vi "AcquireWaveformFromOscill.vi"(4 "error in":errorcluster, 5 "byte count":u32=15000, 6 "Channel (1: Channel 1)":u16(ring)=1 items=["Channel 1"=1, "Channel 2"=2, "Channel 3"=3, "Channel 4"=4], 7 "VISA resource name":refnum<visa-resource-name>) -> (0 "error out":errorcluster, 1 "Number of points":dbl, 2 "Numeric":dbl, 3 "Waveform Graph":waveform(dbl)(graph))   [LabVIEW 2013]
panel:
  out "read buffer":string
  out "Xref":dbl
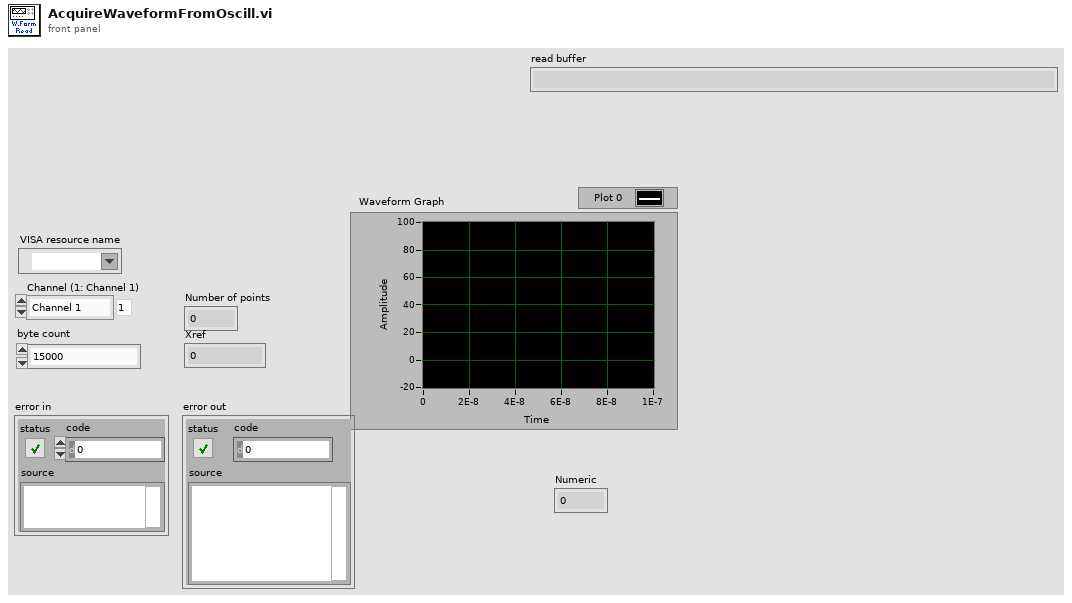
[diagram p1: front panel]
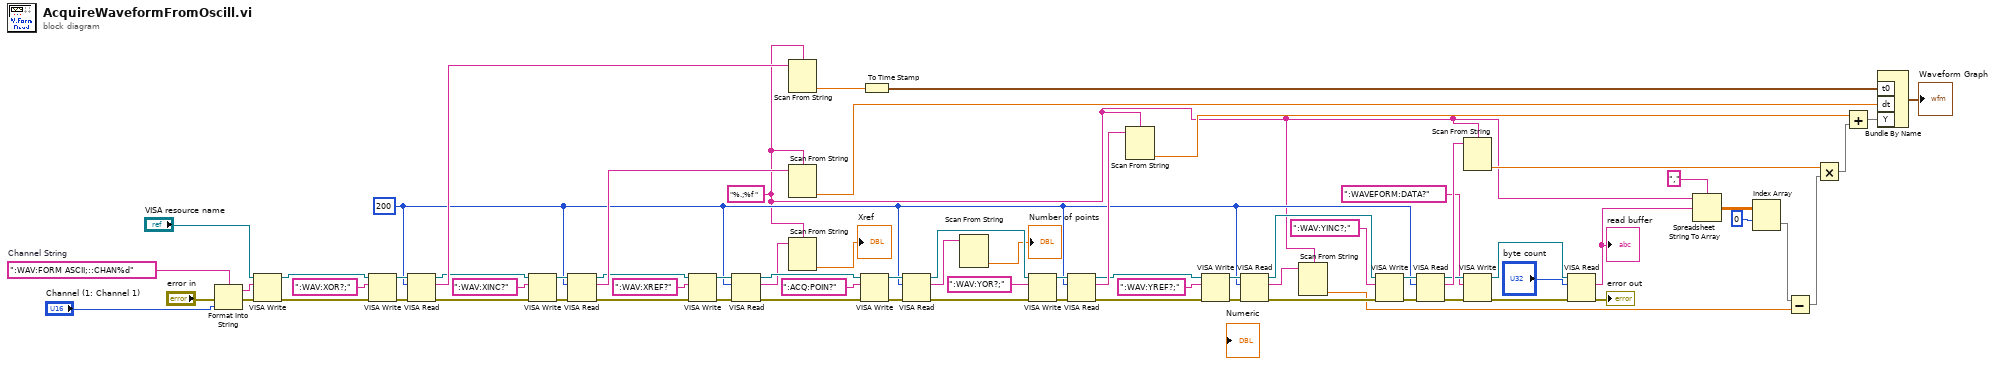
[diagram p0: block diagram]
diagram:
  w9 = ":WAV:FORM ASCII;::CHAN%d"  # Channel String
  w37 = u32 200 ("byte count")
  w12 = "%.;%f " ("format string")
  n1 = Format Into String(format string=w9, error in="error in", "Channel (1: Channel 1)") -> (resulting string=w8:string, error out=w6:errorcluster)  [unwired: 1 in]
  n2 = VISA Write(VISA resource name="VISA resource name", write buffer=w8, error in (no error)=w6) -> (VISA resource name out=w15:refnum<visa-resource-name>, error out=w14:errorcluster)  [unwired: 1 out]
  n3 = VISA Write(VISA resource name=w15, write buffer=":WAV:XOR?;", error in (no error)=w14) -> (VISA resource name out=w74:refnum<visa-resource-name>, error out=w73:errorcluster)  [unwired: 1 out]
  n4 = VISA Read(VISA resource name=w74, byte count=w37, error in (no error)=w73) -> (VISA resource name out=w69:refnum<visa-resource-name>, read buffer=w71:string, error out=w70:errorcluster)  [unwired: 1 out]
  n5 = VISA Write(VISA resource name=w69, write buffer=":WAV:XINC?", error in (no error)=w70) -> (VISA resource name out=w68:refnum<visa-resource-name>, error out=w67:errorcluster)  [unwired: 1 out]
  n6 = VISA Read(VISA resource name=w68, byte count=w37, error in (no error)=w67) -> (VISA resource name out=w55:refnum<visa-resource-name>, read buffer=w66:string, error out=w53:errorcluster)  [unwired: 1 out]
  n7 = VISA Write(VISA resource name=w55, write buffer=":WAV:XREF?", error in (no error)=w53) -> (VISA resource name out=w54:refnum<visa-resource-name>, error out=w52:errorcluster)  [unwired: 1 out]
  n8 = VISA Read(VISA resource name=w54, byte count=w37, error in (no error)=w52) -> (VISA resource name out=w51:refnum<visa-resource-name>, read buffer=w47:string, error out=w50:errorcluster)  [unwired: 1 out]
  n9 = Scan From String(format string=w12, input string=w71) -> (output 1=w26:dbl)  [unwired: 3 in, 3 out]
  n10 = Scan From String(format string=w12, input string=w66) -> (output 1=w1:dbl)  [unwired: 3 in, 3 out]
  n11 = Scan From String(format string=w12, input string=w47) -> (output 1=→"Xref":dbl)  [unwired: 3 in, 3 out]
  n12 = VISA Write(VISA resource name=w51, write buffer=":ACQ:POIN?", error in (no error)=w50) -> (VISA resource name out=w64:refnum<visa-resource-name>, error out=w63:errorcluster)  [unwired: 1 out]
  n13 = To Time Stamp(1:w26) -> (0:w27:timestamp)
  n14 = VISA Read(VISA resource name=w64, byte count=w37, error in (no error)=w63) -> (VISA resource name out=w58:refnum<visa-resource-name>, read buffer=w62:string, error out=w57:errorcluster)  [unwired: 1 out]
  n15 = Scan From String(input string=w62) -> (output 1=→"Number of points":dbl)  [unwired: 4 in, 3 out]
  n16 = VISA Write(VISA resource name=w58, write buffer=":WAV:YOR?;", error in (no error)=w57) -> (VISA resource name out=w61:refnum<visa-resource-name>, error out=w60:errorcluster)  [unwired: 1 out]
  n17 = VISA Read(VISA resource name=w61, byte count=w37, error in (no error)=w60) -> (VISA resource name out=w44:refnum<visa-resource-name>, read buffer=w56:string, error out=w45:errorcluster)  [unwired: 1 out]
  n18 = Scan From String(format string=w12, input string=w56) -> (output 1=w24:dbl)  [unwired: 3 in, 3 out]
  n19 = VISA Write(VISA resource name=w44, write buffer=":WAV:YREF?;", error in (no error)=w45) -> (VISA resource name out=w43:refnum<visa-resource-name>, error out=w46:errorcluster)  [unwired: 1 out]
  n20 = VISA Read(VISA resource name=w43, byte count=w37, error in (no error)=w46) -> (VISA resource name out=w39:refnum<visa-resource-name>, read buffer=w41:string, error out=w36:errorcluster)  [unwired: 1 out]
  n21 = Scan From String(format string=w12, input string=w41) -> (output 1=w25:dbl)  [unwired: 3 in, 3 out]
  n22 = VISA Write(VISA resource name=w39, write buffer=":WAV:YINC?;", error in (no error)=w36) -> (VISA resource name out=w38:refnum<visa-resource-name>, error out=w40:errorcluster)  [unwired: 1 out]
  n23 = VISA Read(VISA resource name=w38, byte count=w37, error in (no error)=w40) -> (VISA resource name out=w32:refnum<visa-resource-name>, read buffer=w34:string, error out=w31:errorcluster)  [unwired: 1 out]
  n24 = Scan From String(format string=w12, input string=w34) -> (output 1=w22:dbl)  [unwired: 3 in, 3 out]
  n25 = VISA Write(VISA resource name=w32, write buffer=":WAVEFORM:DATA?", error in (no error)=w31) -> (VISA resource name out=w29:refnum<visa-resource-name>, error out=w33:errorcluster)  [unwired: 1 out]
  n26 = VISA Read(VISA resource name=w29, byte count="byte count", error in (no error)=w33) -> (read buffer=w20:string, error out=→"error out":errorcluster)  [unwired: 2 out]
  "read buffer" <- w20
  n27 = Spreadsheet String To Array(delimiter (Tab)=",", format string=w12, spreadsheet string=w20) -> (array=w18:dbl[][])  [unwired: 1 in]
  n28 = Index Array(array=w18, index (row)=0) -> (element=w16:dbl[])  [unwired: 1 in]
  n29 = Subtract(x=w16, y=w25) -> (x-y=w23:dbl[])
  n30 = Multiply(x=w22, y=w23) -> (x*y=w3:dbl[])
  n31 = Add(x=w24, y=w3) -> (x+y=w2:dbl[])
  n32 = Bundle By Name ("Build Waveform")("t0"=w27, "dt"=w1, "Y"=w2) -> (→"Waveform Graph":waveform(dbl))  [unwired: 1 in]
